vi "UpdateAccessListTable.vi"(4 "error in (no error)":errorcluster, 6 "id":string, 7 "ADODB._Connection In":refnum<k7>) -> (0 "error out":errorcluster, 3 "ADODB._Connection Out":refnum<k7>)   [LabVIEW 2010]
doc: "This example opens a connection to a database specified by the Connection string (replace the DNS name with your database) inserts a new row into the table \"myOtherTable\" (replace the SQL string with your own SQL query)."
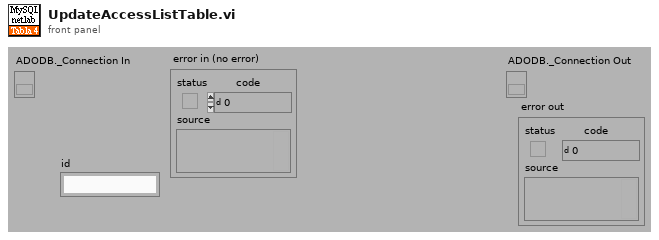
[diagram p1: front panel]
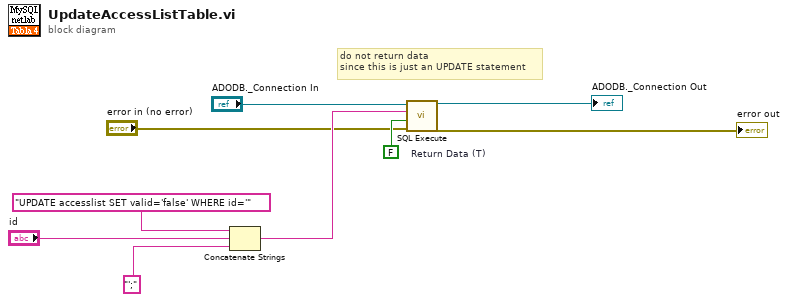
[diagram p0: block diagram]
diagram:
  w7 = FALSE  # Return Data (T)
  # "do not return data\nsince this is just an UPDATE statement"
  n1 = Concatenate Strings("UPDATE accesslist SET valid='false' WHERE id='" ("string"), "id", "';" ("string")) -> (w3:string)
  n2 = call "SQL Execute.vi"("error in (no error)"="error in (no error)", "Return Data (T)"=w7, "Command Text"=w3, "ADODB._Connection In"="ADODB._Connection In") -> ("error out"=→"error out":errorcluster, "ADODB._Connection Out"=→"ADODB._Connection Out":refnum<k7>)  [unwired: 6 out]
